vi "AIT 1553 - Parse BC Sysdef Tree Messages.vi"(8 "error in":errorcluster, 9 "BC Messages In":T2[](array[typedef]), 10 "Section Ptr":T1 format="%.0x") -> (0 "error out":errorcluster, 1 "BC Messages Out":T2[](array[typedef]))   [LabVIEW 2013]
uses:
  <vilib>/NI Veristand/Custom Device API/Custom Device Item Ref.ctl
  Controls/1553_BC_Message.ctl
  Controls/664 -Param.ctl
  Controls and Global/Global.vi
  <vilib>/NI Veristand/Custom Device Tools/Custom Device Utility Library/NI VeriStand - Search for Item by Name.vi
  <vilib>/NI Veristand/Custom Device API/Get Item Property (I32).vi
  <vilib>/NI Veristand/Custom Device API/Get Item Property (Double).vi
  <vilib>/NI Veristand/Custom Device API/Get Item Property (Boolean).vi
  <vilib>/NI Veristand/Custom Device API/Custom Device API.lvlib
  AIT 664 Custom Device.lvlib
  <vilib>/NI Veristand/Custom Device Tools/Custom Device Utility Library/Custom Device Utility Library.lvlib
panel:
  out "Found":bool[](array[boolean])
  out "Property Names":string[][][](array[string])
  out "Channel Refs":T1[][](array[typedef]) format="%.0x"
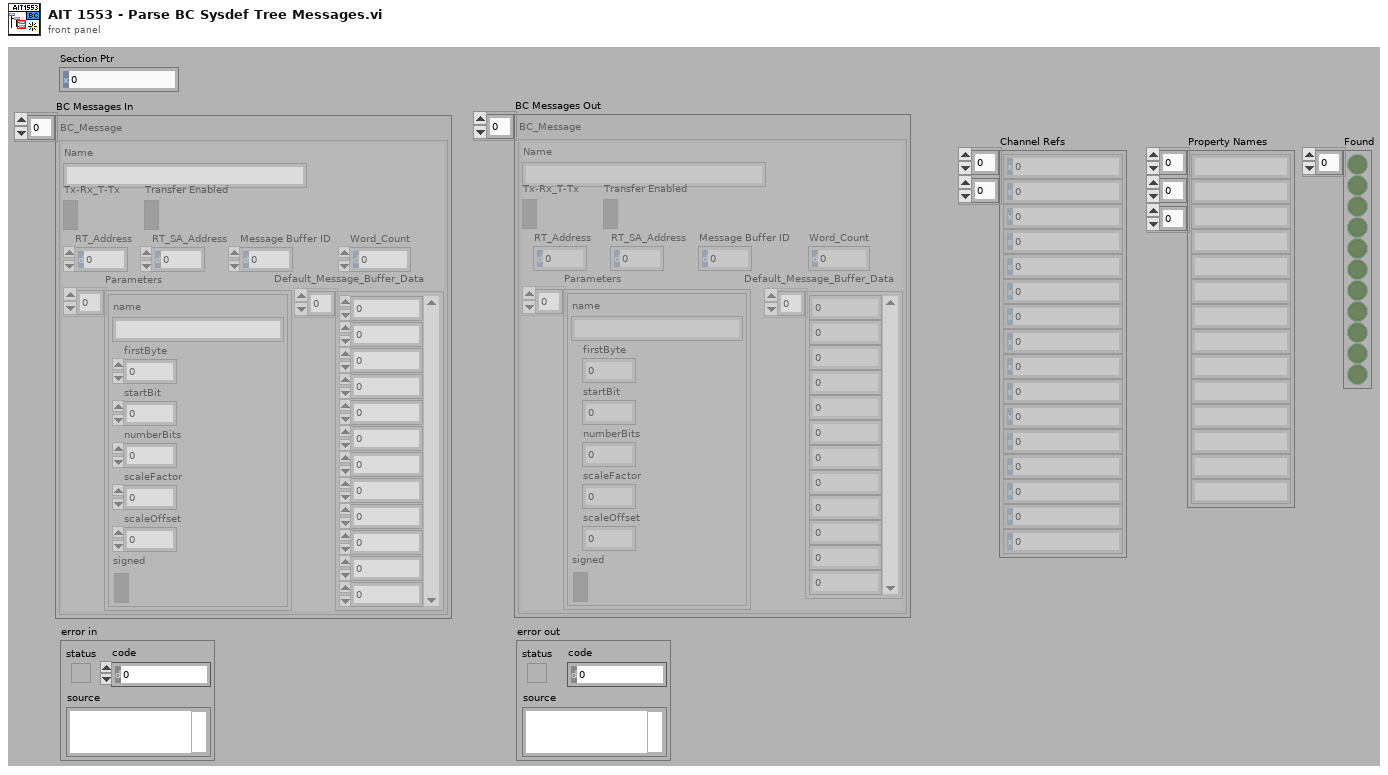
[diagram p1: front panel]
types:
  T1 = typedef "Custom Device API.lvlib/Custom Device Item Ref.ctl" = u64
  T2 = typedef "AIT 664 Custom Device.lvlib/1553_BC_Message.ctl" = cluster{"Name":string, "Tx-Rx_T-Tx":bool, "RT_Address":u8, "RT_SA_Address":u8, "Parameters":T3[], "Transfer Enabled":bool, "Message Buffer ID":u16, "Default_Message_Buffer_Data":u16[], "Word_Count":u8}
  T3 = typedef "AIT 664 Custom Device.lvlib/664 -Param.ctl" = cluster{"name":string, "firstByte":i32, "startBit":i32, "numberBits":i32, "scaleFactor":dbl, "scaleOffset":dbl, "signed":bool}
  T4 = enum32{"Invalid", "Standard", "Closed", "Hidden", "Minimized", "Maximized"}
  T5 = typedef "Custom Device API.lvlib/Custom Device Item Info.ctl" = cluster{"Name":string, "Is Channel":bool, "GUID":string, "Is Waveform":bool}
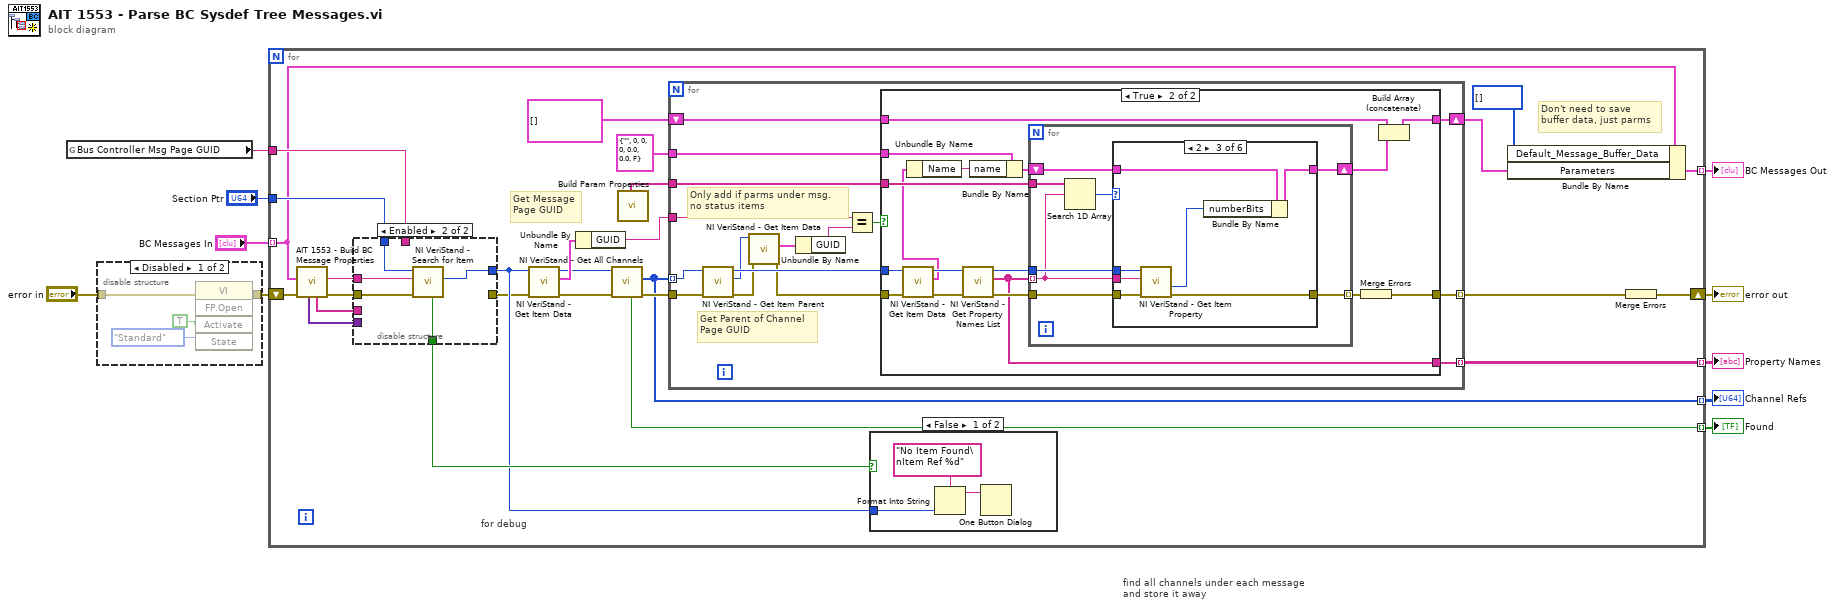
[diagram p0: block diagram]
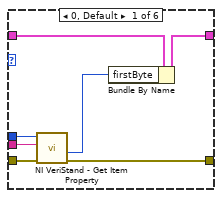
[diagram p5: hidden frame]
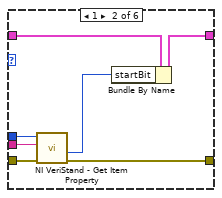
[diagram p6: hidden frame]
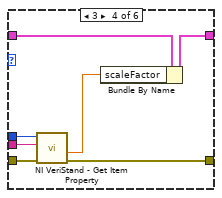
[diagram p7: hidden frame]
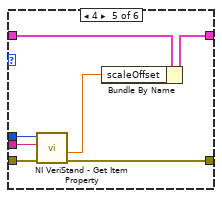
[diagram p8: hidden frame]
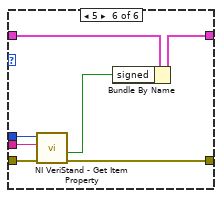
[diagram p9: hidden frame]
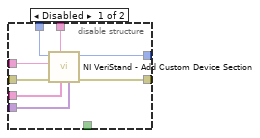
[diagram p10: hidden frame]
diagram:
  # "find all channels under each message\nand store it away"
  n1 = global read "Global.vi" "Bus Controller Msg Page GUID"() -> (w8:string)
  n2 = disable-structure shown="Disabled" {
    disable-tunnel: "error in" -> [w12 w15]
    disable-tunnel: [w11 w15] -> w4
    frame Disabled {
      n3 = invoke class="VI" method="FP.Open"(error in=w12, "Activate"=TRUE ("Activate?"), "State"=T4."Standard") -> (error out=w11:errorcluster)  [unwired: 2 in, 4 out]
    }
    frame Enabled {
    }
  }
  n4 = for {
    shift-right: [w32] -> w10
    shift-left: w4 -> [w38]
    tunnel: "Section Ptr" -> [w36]
    tunnel: "BC Messages In" -> [w31] mode=indexing
    tunnel: w8 -> [w37]
    tunnel: [w30] -> w6 mode=indexing
    tunnel: [w28] -> w3 mode=indexing
    tunnel: [w27] -> w2 mode=indexing
    tunnel: [w26] -> w1 mode=indexing
    # "Get Message\nPage GUID"
    # "Don't need to save\nbuffer data, just parms"
    # "for debug"
    n5 = call "AIT 1553 - Build BC Message Properties.vi"("error in (no error)"=w38, "BC_Message"=w31) -> ("error out"=w40:errorcluster, "name"=w39:string, "Prop Names"=w41:string[], "Prop Values"=w42:variant[])  [unwired: 5 in, 1 out]
    n6 = disable-structure shown="Enabled" {
      disable-tunnel: w42 -> [w138 _]
      disable-tunnel: w41 -> [w137 _]
      disable-tunnel: w40 -> [w136 w142]
      disable-tunnel: w39 -> [w135 w143]
      disable-tunnel: w37 -> [w134 _]
      disable-tunnel: w36 -> [w133 w141]
      disable-tunnel: [w132 _] -> w17
      disable-tunnel: [w131 w140] -> w23
      disable-tunnel: [_ w139] -> w29
      frame Disabled {
        n7 = call <vilib>:"NI VeriStand - Add Custom Device Section.vi"("Property Values"=w138, "Property names"=w137, "GUID (Default Section)"=w134, "error in (no error)"=w136, "Section Name"=w135, "Parent Ref in"=w133) -> ("error out"=w132:errorcluster, "Section Ptr"=w131:T1)  [unwired: 2 in, 2 out]
      }
      frame Enabled {
        n8 = call-poly <vilib>:"NI VeriStand - Search for Item.vi"("error in"=w142, "Item Name"=w143, "Section Ref in"=w141) -> ("Item Ref"=w140:T1, "Found"=w139:bool)  [unwired: 5 in, 2 out]
      }
    }
    n9 = call <vilib>:"NI VeriStand - Get Item Data.vi"("error in (no error)"=w17, "Item Ref in"=w23) -> ("error out"=w16:errorcluster, "Item Info"=w22:T5, "Item Ref out"=w18:T1)  [unwired: 6 in, 1 out]
    n10 = Unbundle By Name(w22) -> ("GUID"=w21:string)
    n11 = call <vilib>:"NI VeriStand - Get All Channels.vi"("error in"=w16, "Section Ref in"=w18) -> ("error out"=w35:errorcluster, "Channel Refs"=w27:T1[], "Found"=w28:bool)  [unwired: 6 in, 1 out]
    n12 = call "Build Param Properties.vi"() -> ("Prop Names"=w34:string[])  [unwired: 11 in, 8 out]
    n13 = for {
      tunnel: w35 -> [w57]
      tunnel: w27 -> [w56] mode=indexing
      tunnel: w34 -> [w61]
      tunnel: [w60] -> w33 mode=indexing
      tunnel: [w58] -> w26 mode=indexing
      tunnel: T3 {"name"="", "firstByte"=0, "startBit"=0, "numberBits"=0, "scaleFactor"=0.0, "scaleOffset"=0.0, "signed"=FALSE} ("1553 Parameter") -> [w59]
      tunnel: w21 -> [w49]
      shift-right: [w46] -> w19
      shift-left: T3[] [] -> [w47]
      # "Only add if parms under msg.\nno status items"
      # "Get Parent of Channel\nPage GUID"
      n14 = call <vilib>:"NI VeriStand - Get Item Parent.vi"("error in (no error)"=w57, "Item Ref in"=w56) -> ("error out"=w54:errorcluster, "Parent Ref"=w52:T1, "Item Ref out"=w55:T1)  [unwired: 6 in, 1 out]
      n15 = call <vilib>:"NI VeriStand - Get Item Data.vi"("error in (no error)"=w54, "Item Ref in"=w52) -> ("error out"=w53:errorcluster, "Item Info"=w51:T5)  [unwired: 6 in, 2 out]
      n16 = Unbundle By Name(w51) -> ("GUID"=w50:string)
      n17 = Equal?(x=w49, y=w50) -> (x = y?=w48:bool)
      n18 = case shown="True" w48 {
        tunnel: w61 -> [_ w79]
        tunnel: [w62 w76] -> w60
        tunnel: w59 -> [_ w73]
        tunnel: [_ w69] -> w58
        tunnel: w55 -> [_ w68]
        tunnel: w53 -> [w62 w67]
        tunnel: w47 -> [w63 w66]
        tunnel: [w63 w64] -> w46
        frame False {
        }
        frame True {
          n19 = call <vilib>:"NI VeriStand - Get Item Data.vi"("error in (no error)"=w67, "Item Ref in"=w68) -> ("error out"=w75:errorcluster, "Item Info"=w70:T5, "Item Ref out"=w74:T1)  [unwired: 6 in, 1 out]
          n20 = Unbundle By Name(w70) -> ("Name"=w71:string)
          n21 = call <vilib>:"NI VeriStand - Get Property Names List.vi"("error in (no error)"=w75, "Item Ref in"=w74) -> ("error out"=w80:errorcluster, "Property Names"=w69:string[], "Item Ref out"=w78:T1)  [unwired: 7 in]
          n22 = Bundle By Name(cluster=w73, "name"=w71) -> (w72:T3)
          n23 = for {
            tunnel: w80 -> [w85]
            tunnel: w69 -> [w83] mode=indexing
            tunnel: w79 -> [w88]
            shift-right: [w82] -> w65
            shift-left: w72 -> [w86]
            tunnel: w78 -> [w84]
            tunnel: [w81] -> w77 mode=indexing
            n24 = Search 1D Array(1D array=w88, element=w83) -> (index of element=w87:i32)  [unwired: 1 in]
            n25 = case shown="2" w87 {
              tunnel: w86 -> [w95 w102 w109 w116 w123 w130]
              tunnel: w85 -> [w94 w101 w108 w115 w122 w129]
              tunnel: w84 -> [w93 w100 w107 w114 w121 w128]
              tunnel: w83 -> [w92 w99 w106 w113 w120 w127]
              tunnel: [w90 w97 w104 w111 w118 w125] -> w82
              tunnel: [w89 w96 w103 w110 w117 w124] -> w81
              frame 0, Default {
                n26 = call-poly <vilib>:"NI VeriStand - Get Item Property.vi"("error in (no error)"=w94, "Property Name"=w92, "Item Ref in"=w93) -> ("error out"=w89:errorcluster, "Value"=w91:i32)  [unwired: 5 in, 2 out]
                n27 = Bundle By Name(cluster=w95, "firstByte"=w91) -> (w90:T3)
              }
              frame 1 {
                n28 = call-poly <vilib>:"NI VeriStand - Get Item Property.vi"("error in (no error)"=w101, "Property Name"=w99, "Item Ref in"=w100) -> ("error out"=w96:errorcluster, "Value"=w98:i32)  [unwired: 5 in, 2 out]
                n29 = Bundle By Name(cluster=w102, "startBit"=w98) -> (w97:T3)
              }
              frame 2 {
                n30 = call-poly <vilib>:"NI VeriStand - Get Item Property.vi"("error in (no error)"=w108, "Property Name"=w106, "Item Ref in"=w107) -> ("error out"=w103:errorcluster, "Value"=w105:i32)  [unwired: 5 in, 2 out]
                n31 = Bundle By Name(cluster=w109, "numberBits"=w105) -> (w104:T3)
              }
              frame 3 {
                n32 = call-poly <vilib>:"NI VeriStand - Get Item Property.vi"("error in (no error)"=w115, "Property Name"=w113, "Item Ref in"=w114) -> ("error out"=w110:errorcluster, "Value"=w112:dbl)  [unwired: 5 in, 2 out]
                n33 = Bundle By Name(cluster=w116, "scaleFactor"=w112) -> (w111:T3)
              }
              frame 4 {
                n34 = call-poly <vilib>:"NI VeriStand - Get Item Property.vi"("error in (no error)"=w122, "Property Name"=w120, "Item Ref in"=w121) -> ("error out"=w117:errorcluster, "Value"=w119:dbl)  [unwired: 5 in, 2 out]
                n35 = Bundle By Name(cluster=w123, "scaleOffset"=w119) -> (w118:T3)
              }
              frame 5 {
                n36 = call-poly <vilib>:"NI VeriStand - Get Item Property.vi"("error in (no error)"=w129, "Property Name"=w127, "Item Ref in"=w128) -> ("error out"=w124:errorcluster, "Value"=w126:bool)  [unwired: 5 in, 2 out]
                n37 = Bundle By Name(cluster=w130, "signed"=w126) -> (w125:T3)
              }
            }
          }
          n38 = Merge Errors(w77) -> (w76:errorcluster)
          n39 = Build Array (concatenate)(w66, w65) -> (w64:T3[])
        }
      }
    }
    n40 = case shown="False" w29 {
      tunnel: w23 -> [w45 _]
      frame False {
        n41 = Format Into String(format string="No Item Found\nItem Ref %d" ("message"), w45) -> (resulting string=w44:string)  [unwired: 2 in, 1 out]
        n42 = One Button Dialog(message=w44) -> ()  [unwired: 1 in, 1 out]
      }
      frame True {
      }
    }
    n43 = Bundle By Name(cluster=w31, "Default_Message_Buffer_Data"=u16[] [], "Parameters"=w19) -> (w30:T2)
    n44 = Merge Errors(w33) -> (w32:errorcluster)
  }
  "error out" <- w10
  "BC Messages Out" <- w6
  "Found" <- w3
  "Channel Refs" <- w2
  "Property Names" <- w1
